vi "Simulated Automotive Data.vi"() -> ()   [LabVIEW 2020]
uses:
  FlexLoggerTagHelpers.lvlib
  <vilib>/Skyline/Tag/Wrapper/Wrapper_class/NI Skyline Tag.lvclass
  <vilib>/Skyline/Tag/Wrapper/Wrapper AMQP_class/Open Tag AMQP.vi
  <vilib>/Skyline/Tag/Wrapper/Wrapper AMQP_class/NI Skyline Tag AMQP.lvclass
  <vilib>/Skyline/Tag/Shared/typedefs/DataType.ctl
  <vilib>/Skyline/Tag/Shared/NI Skyline Tag.lvlib
  <vilib>/Skyline/Tag/Wrapper/Wrapper_class/Write Tag (DBL).vi
  <vilib>/Skyline/Tag/Wrapper/Wrapper_class/Close Tag (Single).vi
  <vilib>/Skyline/Tag/Wrapper/Wrapper_class/Read Tag (DBL).vi
panel:
  out "Odometer":dbl
  out "Automotive Data":T1(graph)
  in  "Stop":bool
  # "Overview: This example shows how to plug in external data to FlexLogger using SystemLink Tags.  Simulated temperature\nreadings from a chamber are written to FlexLogger SystemLink tags at a rate ten updates per second.\nRequirements: LabVIEW Full Development System, FlexLogger\nInstructions:\n1. Launch FlexLogger\n     a. Create a Project.\n     b. Using the Project >> Settings menu, enable Publish SystemLink Tags (Export) and Consume External SystemLink Tags (Import).\n     c. Restart the FlexLogger Project.\n2. Run this VI. \n3. Within the FlexLogger project:\n     a. Note that the new exported tags appear in the Channel Specification page.\n     b. Switch to the Screen document, drop a Long History Graph, and connect the new tag channels to the graph.\n4. Click on the Stop button to stop this VI and close all SystemLink tags.  \n5. Note that in FlexLogger all channels connected to the temperature tags will no longer update."
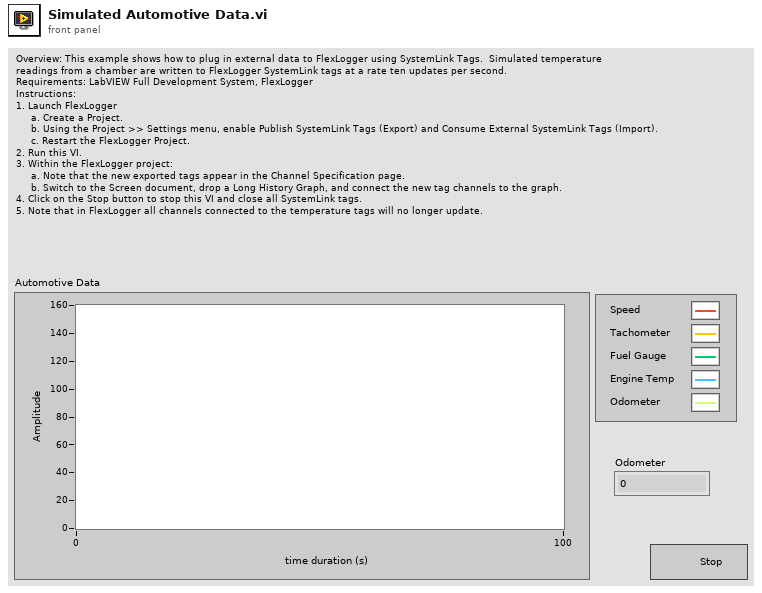
[diagram p1: front panel]
types:
  T1 = cluster{"Speed":dbl, "RPM":dbl, "Fuel Gauge":dbl, "Temperature":dbl, dbl}
  T2 = typedef "NI Skyline Tag.lvlib/DataType.ctl" = enum32{"Double", "I32", "String", "Boolean", "U64", "Timestamp"}
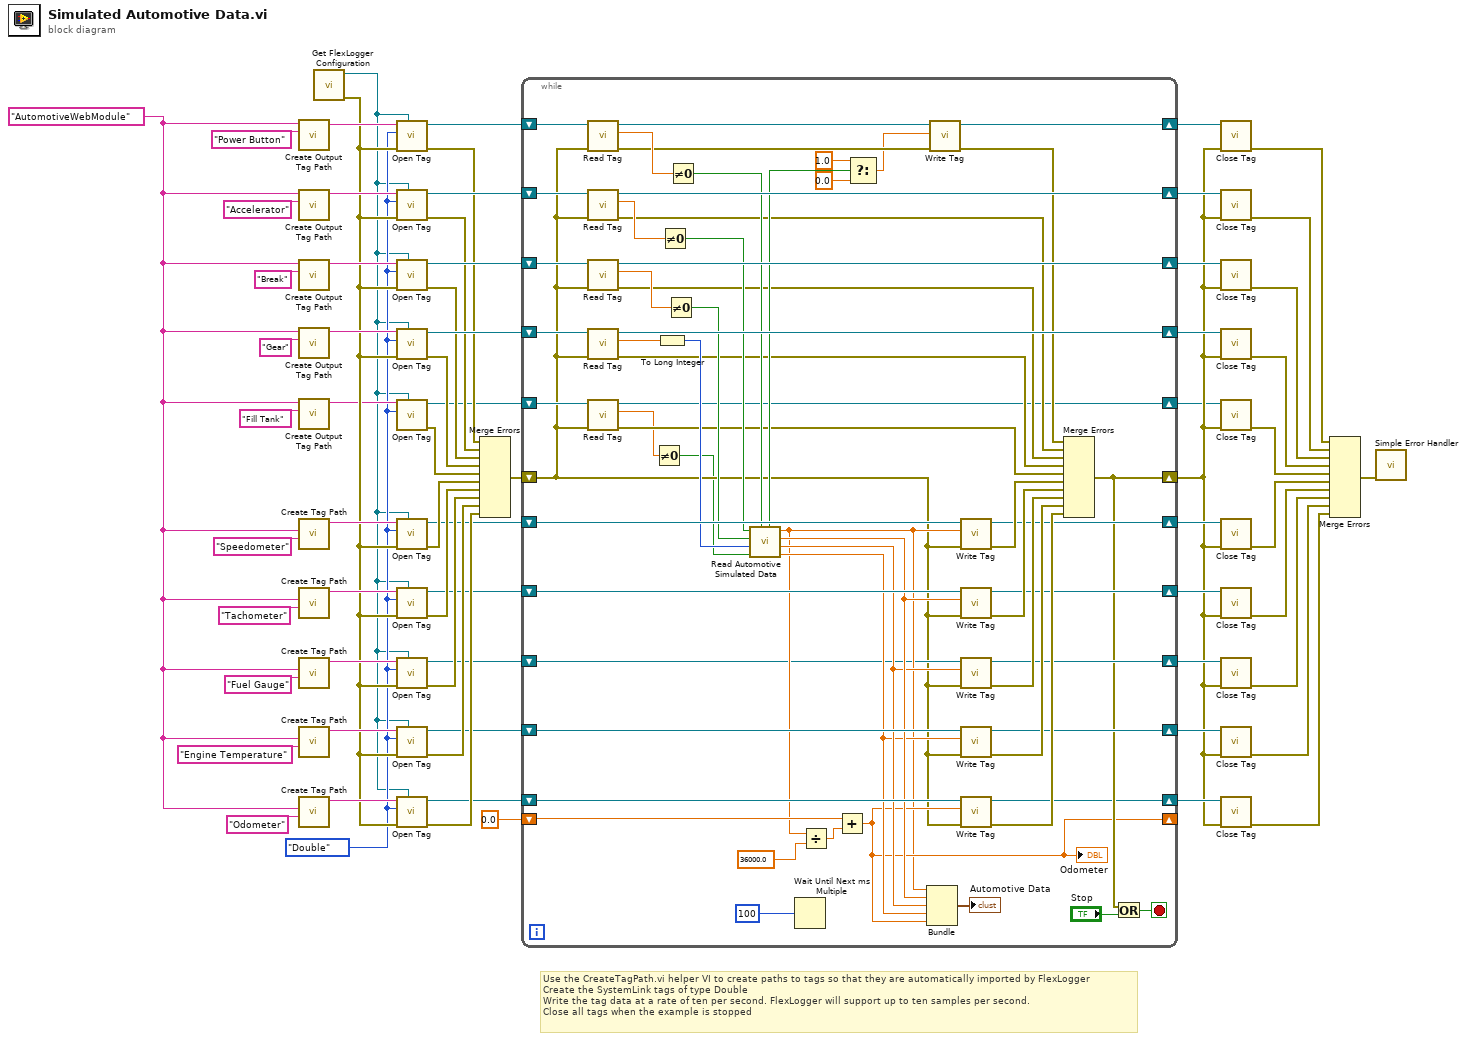
[diagram p0: block diagram]
diagram:
  w5 = DataType."Double" ("data type")
  w9 = "AutomotiveWebModule" ("Group Name")
  # "Use the CreateTagPath.vi helper VI to create paths to tags so that they are automatically imported by FlexLogger\nCreate the SystemLink tags of type Double\nWrite the tag data at a rate of ten per second. FlexLogger will support up to ten samples per second.\nClose all tags when the example is stopped"
  n1 = call "Create Output Tag Path.vi"("Channel Name"="Power Button", "Group Name"=w9) -> ("Path"=w28:string)  [unwired: 9 in]
  n2 = call "Create Output Tag Path.vi"("Channel Name"="Accelerator", "Group Name"=w9) -> ("Path"=w29:string)  [unwired: 9 in]
  n3 = call "Create Output Tag Path.vi"("Channel Name"="Break", "Group Name"=w9) -> ("Path"=w30:string)  [unwired: 9 in]
  n4 = call "Create Output Tag Path.vi"("Channel Name"="Gear", "Group Name"=w9) -> ("Path"=w31:string)  [unwired: 9 in]
  n5 = call "Create Output Tag Path.vi"("Channel Name"="Fill Tank", "Group Name"=w9) -> ("Path"=w8:string)  [unwired: 9 in]
  n6 = call "Create Tag Path.vi"("channel name"="Speedometer" ("Channel Name"), "group name"=w9) -> ("tag path"=w62:string)  [unwired: 9 in]
  n7 = call "Create Tag Path.vi"("channel name"="Tachometer" ("Channel Name"), "group name"=w9) -> ("tag path"=w61:string)  [unwired: 9 in]
  n8 = call "Create Tag Path.vi"("channel name"="Fuel Gauge" ("Channel Name"), "group name"=w9) -> ("tag path"=w60:string)  [unwired: 9 in]
  n9 = call "Create Tag Path.vi"("channel name"="Engine Temperature" ("Channel Name"), "group name"=w9) -> ("tag path"=w59:string)  [unwired: 9 in]
  n10 = call "Create Tag Path.vi"("channel name"="Odometer" ("Channel Name"), "group name"=w9) -> ("tag path"=w58:string)  [unwired: 9 in]
  n11 = call "Get FlexLogger Configuration.vi"() -> ("error out"=w27:errorcluster, "Local FlexLogger Configuration"=w4:refnum<class "NI Skyline Configuration AMQP.lvclass">)  [unwired: 10 in]
  n12 = call-poly <vilib>:"Open Tag.vi"("configuration"=w4, "error in (no error)"=w27, "data type"=w5, "path"=w28) -> ("error out"=w14:errorcluster, "tag"=w26:refnum<class "NI Skyline Tag.lvclass">)  [unwired: 6 in]
  n13 = call-poly <vilib>:"Open Tag.vi"("configuration"=w4, "error in (no error)"=w27, "data type"=w5, "path"=w29) -> ("error out"=w13:errorcluster, "tag"=w24:refnum<class "NI Skyline Tag.lvclass">)  [unwired: 6 in]
  n14 = call-poly <vilib>:"Open Tag.vi"("configuration"=w4, "error in (no error)"=w27, "data type"=w5, "path"=w30) -> ("error out"=w12:errorcluster, "tag"=w22:refnum<class "NI Skyline Tag.lvclass">)  [unwired: 6 in]
  n15 = call-poly <vilib>:"Open Tag.vi"("configuration"=w4, "error in (no error)"=w27, "data type"=w5, "path"=w31) -> ("error out"=w11:errorcluster, "tag"=w20:refnum<class "NI Skyline Tag.lvclass">)  [unwired: 6 in]
  n16 = call-poly <vilib>:"Open Tag.vi"("configuration"=w4, "data type"=w5, "path"=w8) -> ("error out"=w6:errorcluster, "tag"=w7:refnum<class "NI Skyline Tag.lvclass">)  [unwired: 7 in]
  n17 = call-poly <vilib>:"Open Tag.vi"("configuration"=w4, "error in (no error)"=w27, "data type"=w5, "path"=w62) -> ("error out"=w56:errorcluster, "tag"=w37:refnum<class "NI Skyline Tag.lvclass">)  [unwired: 6 in]
  n18 = call-poly <vilib>:"Open Tag.vi"("configuration"=w4, "error in (no error)"=w27, "data type"=w5, "path"=w61) -> ("error out"=w55:errorcluster, "tag"=w50:refnum<class "NI Skyline Tag.lvclass">)  [unwired: 6 in]
  n19 = call-poly <vilib>:"Open Tag.vi"("configuration"=w4, "error in (no error)"=w27, "data type"=w5, "path"=w60) -> ("error out"=w57:errorcluster, "tag"=w48:refnum<class "NI Skyline Tag.lvclass">)  [unwired: 6 in]
  n20 = call-poly <vilib>:"Open Tag.vi"("configuration"=w4, "error in (no error)"=w27, "data type"=w5, "path"=w59) -> ("error out"=w54:errorcluster, "tag"=w46:refnum<class "NI Skyline Tag.lvclass">)  [unwired: 6 in]
  n21 = call-poly <vilib>:"Open Tag.vi"("configuration"=w4, "error in (no error)"=w27, "data type"=w5, "path"=w58) -> ("error out"=w53:errorcluster, "tag"=w44:refnum<class "NI Skyline Tag.lvclass">)  [unwired: 6 in]
  n22 = Merge Errors(w14, w13, w12, w11, w6, w56, w55, w57, w54, w53) -> (w52:errorcluster)
  n23 = while {
    shift-right: [w121] -> w51
    shift-left: w37 -> [w112]
    shift-right: [w119] -> w49
    shift-left: w50 -> [w120]
    shift-right: [w118] -> w47
    shift-left: w48 -> [w79]
    shift-right: [w116] -> w45
    shift-left: w46 -> [w117]
    shift-right: [w111] -> w43
    shift-left: w44 -> [w115]
    shift-right: [w114] -> w2
    shift-left: w52 -> [w77]
    shift-right: [w105] -> _
    shift-left: 0.0 -> [w110]
    shift-right: [w95] -> w19
    shift-left: w20 -> [w96]
    shift-right: [w97] -> w21
    shift-left: w22 -> [w98]
    shift-right: [w99] -> w23
    shift-left: w24 -> [w100]
    shift-right: [w85] -> w25
    shift-left: w26 -> [w101]
    shift-right: [w71] -> w1
    shift-left: w7 -> [w78]
    stop <- w128 stop-if-true
    n24 = call-poly <vilib>:"Read Tag.vi"("error in (no error)"=w77, "tag in"=w101) -> ("error out"=w84:errorcluster, "value"=w94:dbl, "tag out"=w86:refnum<class "NI Skyline Tag.lvclass">)  [unwired: 5 in, 2 out]
    n25 = call-poly <vilib>:"Read Tag.vi"("error in (no error)"=w77, "tag in"=w100) -> ("error out"=w75:errorcluster, "value"=w92:dbl, "tag out"=w99:refnum<class "NI Skyline Tag.lvclass">)  [unwired: 5 in, 2 out]
    n26 = call-poly <vilib>:"Read Tag.vi"("error in (no error)"=w77, "tag in"=w98) -> ("error out"=w74:errorcluster, "value"=w90:dbl, "tag out"=w97:refnum<class "NI Skyline Tag.lvclass">)  [unwired: 5 in, 2 out]
    n27 = call-poly <vilib>:"Read Tag.vi"("error in (no error)"=w77, "tag in"=w96) -> ("error out"=w73:errorcluster, "value"=w88:dbl, "tag out"=w95:refnum<class "NI Skyline Tag.lvclass">)  [unwired: 5 in, 2 out]
    n28 = call-poly <vilib>:"Read Tag.vi"("error in (no error)"=w77, "tag in"=w78) -> ("error out"=w72:errorcluster, "value"=w70:dbl, "tag out"=w71:refnum<class "NI Skyline Tag.lvclass">)  [unwired: 5 in, 2 out]
    n29 = Not Equal To 0?(x=w70) -> (x != 0?=w69:bool)
    n30 = To Long Integer(number=w88) -> (32bit integer=w87:i32)
    n31 = Not Equal To 0?(x=w92) -> (x != 0?=w91:bool)
    n32 = Not Equal To 0?(x=w90) -> (x != 0?=w89:bool)
    n33 = Not Equal To 0?(x=w94) -> (x != 0?=w93:bool)
    n34 = call "Read Automotive Simulated Data.vi"("Power Button"=w93, 8:w69, "Gear"=w87, "Break"=w89, "Accelerator"=w91) -> ("Temperature"=w106:dbl, "Fuel Gauge"=w107:dbl, "RPM"=w108:dbl, "Speed"=w104:dbl, "ON"=w83:bool)  [unwired: 2 in]
    n35 = Wait Until Next ms Multiple(millisecond multiple=u32 100 ("milliseconds to wait")) -> ()  [unwired: 1 out]
    n36 = Divide(x=w104, y=36000.0 ("x")) -> (x/y=w102:dbl)
    n37 = Add(x=w110, y=w102) -> (x+y=w105:dbl)
    "Odometer" <- w105
    n38 = Select(t=1.0, s=w83, f=0.0) -> (s? t:f=w80:dbl)
    n39 = Bundle("Speed"=w104, "RPM"=w108, "Fuel Gauge"=w107, "Temperature"=w106, w105) -> (→"Automotive Data":T1)  [unwired: 1 in]
    n40 = call-poly <vilib>:"Write Tag.vi"("error in (no error)"=w84, "value"=w80, "tag in"=w86) -> ("error out"=w76:errorcluster, "tag out"=w85:refnum<class "NI Skyline Tag.lvclass">)  [unwired: 7 in]
    n41 = call-poly <vilib>:"Write Tag.vi"("error in (no error)"=w77, "value"=w104, "tag in"=w112) -> ("error out"=w126:errorcluster, "tag out"=w121:refnum<class "NI Skyline Tag.lvclass">)  [unwired: 7 in]
    n42 = call-poly <vilib>:"Write Tag.vi"("error in (no error)"=w77, "value"=w108, "tag in"=w120) -> ("error out"=w124:errorcluster, "tag out"=w119:refnum<class "NI Skyline Tag.lvclass">)  [unwired: 7 in]
    n43 = call-poly <vilib>:"Write Tag.vi"("error in (no error)"=w77, "value"=w107, "tag in"=w79) -> ("error out"=w125:errorcluster, "tag out"=w118:refnum<class "NI Skyline Tag.lvclass">)  [unwired: 7 in]
    n44 = call-poly <vilib>:"Write Tag.vi"("error in (no error)"=w77, "value"=w106, "tag in"=w117) -> ("error out"=w123:errorcluster, "tag out"=w116:refnum<class "NI Skyline Tag.lvclass">)  [unwired: 7 in]
    n45 = call-poly <vilib>:"Write Tag.vi"("error in (no error)"=w77, "value"=w105, "tag in"=w115) -> ("error out"=w122:errorcluster, "tag out"=w111:refnum<class "NI Skyline Tag.lvclass">)  [unwired: 7 in]
    n46 = Merge Errors(w76, w75, w74, w73, w72, w126, w124, w125, w123, w122) -> (w114:errorcluster)
    n47 = Or(x=w114, y="Stop") -> (x .or. y?=w128:bool)
  }
  n48 = call-poly <vilib>:"Close Tag.vi"("error in (no error)"=w2, "tag"=w25) -> ("error out"=w18:errorcluster)  [unwired: 9 in]
  n49 = call-poly <vilib>:"Close Tag.vi"("error in (no error)"=w2, "tag"=w23) -> ("error out"=w17:errorcluster)  [unwired: 9 in]
  n50 = call-poly <vilib>:"Close Tag.vi"("error in (no error)"=w2, "tag"=w21) -> ("error out"=w16:errorcluster)  [unwired: 9 in]
  n51 = call-poly <vilib>:"Close Tag.vi"("error in (no error)"=w2, "tag"=w19) -> ("error out"=w15:errorcluster)  [unwired: 9 in]
  n52 = call-poly <vilib>:"Close Tag.vi"("error in (no error)"=w2, "tag"=w1) -> ("error out"=w3:errorcluster)  [unwired: 9 in]
  n53 = call-poly <vilib>:"Close Tag.vi"("error in (no error)"=w2, "tag"=w51) -> ("error out"=w42:errorcluster)  [unwired: 9 in]
  n54 = call-poly <vilib>:"Close Tag.vi"("error in (no error)"=w2, "tag"=w49) -> ("error out"=w41:errorcluster)  [unwired: 9 in]
  n55 = call-poly <vilib>:"Close Tag.vi"("error in (no error)"=w2, "tag"=w47) -> ("error out"=w40:errorcluster)  [unwired: 9 in]
  n56 = call-poly <vilib>:"Close Tag.vi"("error in (no error)"=w2, "tag"=w45) -> ("error out"=w39:errorcluster)  [unwired: 9 in]
  n57 = call-poly <vilib>:"Close Tag.vi"("error in (no error)"=w2, "tag"=w43) -> ("error out"=w38:errorcluster)  [unwired: 9 in]
  n58 = Merge Errors(w18, w17, w16, w15, w3, w42, w41, w40, w39, w38) -> (w65:errorcluster)
  n59 = call <vilib>:"Simple Error Handler.vi"("error in (no error)"=w65) -> ()  [unwired: 4 in, 5 out]
